vi "Siglent SDS 1000 2000 Series Acquire Multiple Waveforms.vi"() -> ()   [LabVIEW 2021]
doc: "This example shows how to configure multiple channels and acquire waveforms from multiple channels."
uses:
  <instrlib>/Siglent SDS 1000 2000 Series/Public/Data/Read Waveform (Multiple).vi
  <instrlib>/Siglent SDS 1000 2000 Series/Siglent SDS 1000 2000 Series.lvlib
panel:
  in  "Channel (2: Channel 2)":u16(ring)=2 items=["Channel 1"=1, "Channel 2"=2, "Channel 3"=3, "Channel 4"=4]
  in  "Channel (1: Channel 1)":u16(ring)=1 items=["Channel 1"=1, "Channel 2"=2, "Channel 3"=3, "Channel 4"=4]
  in  "Vertical Coupling (0: A1M)":u16(ring) items=["A1M", "A50", "D1M", "D50", "Ground"]
  in  "Vertical Coupling (0: A1M)":u16(ring) items=["A1M", "A50", "D1M", "D50", "Ground"]
  in  "Vertical Offset (0.0 V)":dbl
  in  "Vertical Offset (0.0 V)":dbl
  in  "Probe Attenuation (1X)":dbl=1.0
  in  "Probe Attenuation (1X)":dbl=1.0
  in  "Timeout (10000 ms)":u32=10000
  out "Waveform Data":waveform(dbl)[](graph)
  in  "VISA resource name":refnum<visa-resource-name>
  # "(c) 2015 SIGLENT TECHNOLOGIES CO., LTD.   ALL RIGHTS RESERVED."
  # "Channel A"
  # "Channel B"
  # "Note:\nThis VI will time out without acquiring any data if the input signal on the selected channel does not cross 0 V trigger level with positive slope."
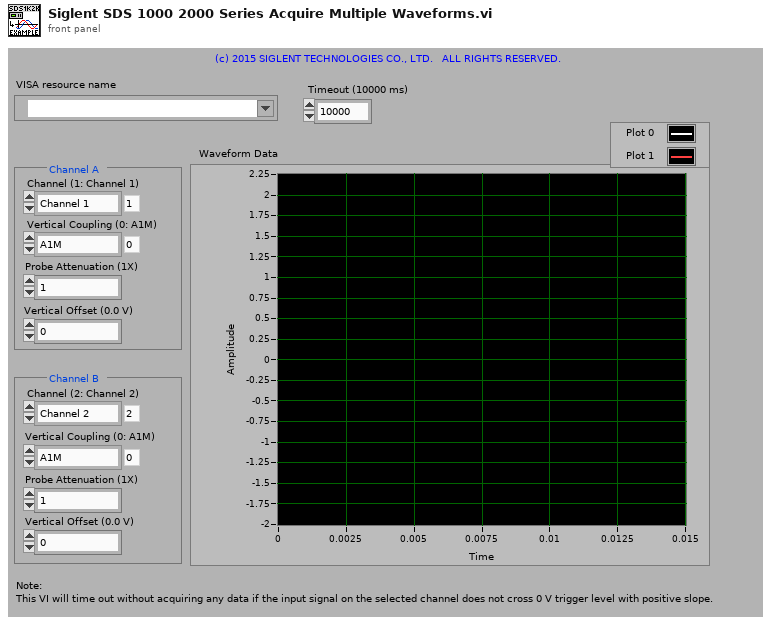
[diagram p1: front panel]
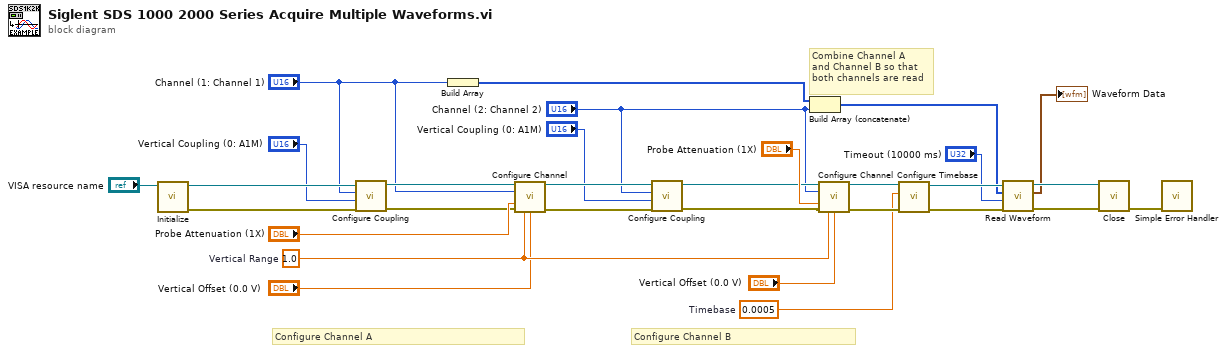
[diagram p0: block diagram]
diagram:
  w20 = 1.0  # Vertical Range
  w19 = 0.0005  # Timebase
  # "Combine Channel A\nand Channel B so that\nboth channels are read"
  # "Configure Channel B"
  # "Configure Channel A"
  n1 = call <instrlib>:"Initialize.vi"("VISA resource name"="VISA resource name") -> ("error out"=w4:errorcluster, "VISA resource name out"=w6:refnum<visa-resource-name>)  [unwired: 9 in]
  n2 = call <instrlib>:"Configure Coupling.vi"("error in (no error)"=w4, "Vertical Coupling (0: A1M)"="Vertical Coupling (0: A1M)", "Channel (1: Channel 1)"="Channel (1: Channel 1)", "VISA resource name"=w6) -> ("error out"=w3:errorcluster, "VISA resource name out"=w5:refnum<visa-resource-name>)  [unwired: 6 in]
  n3 = Build Array("Channel (1: Channel 1)") -> (w15:u16[])
  n4 = call <instrlib>:"Configure Channel.vi"("VISA resource name"=w5, "Channel (1: Channel 1)"="Channel (1: Channel 1)", "Probe Attenuation (1X)"="Probe Attenuation (1X)", "error in (no error)"=w3, "Vertical Range (1.0 V)"=w20, "Vertical Offset (0.0 V)"="Vertical Offset (0.0 V)") -> ("VISA resource name out"=w12:refnum<visa-resource-name>, "error out"=w11:errorcluster)  [unwired: 8 in]
  n5 = call <instrlib>:"Configure Coupling.vi"("error in (no error)"=w11, "Vertical Coupling (0: A1M)"="Vertical Coupling (0: A1M)", "Channel (1: Channel 1)"="Channel (2: Channel 2)", "VISA resource name"=w12) -> ("error out"=w9:errorcluster, "VISA resource name out"=w10:refnum<visa-resource-name>)  [unwired: 6 in]
  n6 = Build Array (concatenate)(w15, "Channel (2: Channel 2)") -> (w14:u16[])
  n7 = call <instrlib>:"Configure Channel.vi"("VISA resource name"=w10, "Channel (1: Channel 1)"="Channel (2: Channel 2)", "Probe Attenuation (1X)"="Probe Attenuation (1X)", "error in (no error)"=w9, "Vertical Range (1.0 V)"=w20, "Vertical Offset (0.0 V)"="Vertical Offset (0.0 V)") -> ("VISA resource name out"=w26:refnum<visa-resource-name>, "error out"=w25:errorcluster)  [unwired: 8 in]
  n8 = call <instrlib>:"Configure Timebase.vi"("error in (no error)"=w25, "Timebase (0.0005 s)"=w19, "VISA resource name"=w26) -> ("error out"=w23:errorcluster, "VISA resource name out"=w24:refnum<visa-resource-name>)  [unwired: 7 in]
  n9 = call-poly <instrlib>:"Read Waveform.vi"("error in (no error)"=w23, "Timeout (10000 ms)"="Timeout (10000 ms)", "Channels"=w14, "VISA resource name"=w24) -> ("error out"=w27:errorcluster, "Waveform Data"=→"Waveform Data":waveform(dbl)[], "VISA resource name out"=w28:refnum<visa-resource-name>)  [unwired: 5 in]
  n10 = call <instrlib>:"Close.vi"("error in (no error)"=w27, "VISA resource name"=w28) -> ("error out"=w29:errorcluster)  [unwired: 9 in]
  n11 = call <vilib>:"Simple Error Handler.vi"("error in (no error)"=w29) -> ()  [unwired: 4 in, 5 out]
